vi "Connection State Callback.vi"(7 "Owner":refnum<class>, 8 "error in (no error)":errorcluster, 10 "Connection State":T1, 11 "Connection":refnum<class "Connection.lvclass">) -> (0 "error out":errorcluster)   [LabVIEW 2012, in "Chat Server.lvclass"]
uses:
  Chat Server.lvclass
  lv-stream/stream/Connection/Connection.lvclass
  lv-stream/stream/Connection State.ctl
  lv-stream/stream/Stream.lvlib
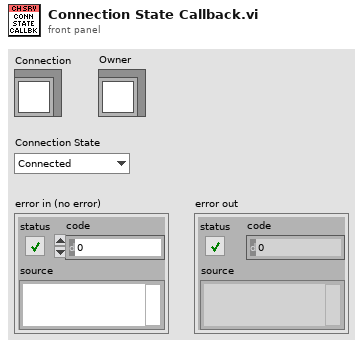
[diagram p1: front panel]
types:
  T1 = typedef "Stream.lvlib/Connection State.ctl" = enum16{"Connected", "Disconnected"}
  T2 = typedef "Chat Server.lvclass/Red Data.ctl" = cluster{"Connections":refnum<class "Connection.lvclass">[]}
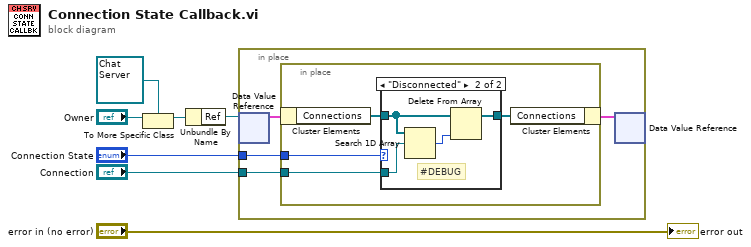
[diagram p0: block diagram]
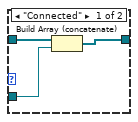
[diagram p2: hidden frame]
diagram:
  n1 = To More Specific Class(target class=refnum<class "Chat Server.lvclass"> refnum ("Chat Server.lvclass"), reference="Owner") -> (specific class reference=w4:refnum<class "Chat Server.lvclass">)  [unwired: 1 in, 1 out]
  n2 = Unbundle By Name(w4) -> ("Ref"=w5:refnum<data-value>)
  n3 = in-place {
    in-place-border: "Connection" -> [w9]
    in-place-border: "Connection State" -> [w8]
    n4 = in-place-dvr #1(w5) -> (w11:T2)  [unwired: 1 out]
    n5 = in-place {
      in-place-border: w9 -> [w13]
      in-place-border: w8 -> [w15]
      n6 = in-place-cluster #2(w11) -> ("Connections"=w14:refnum<class "Connection.lvclass">[])
      n7 = case shown="\"Disconnected\"" w15 {
        tunnel: w14 -> [w18 w21]
        tunnel: w13 -> [w17 w22]
        tunnel: [w16 w19] -> w12
        frame "Connected" {
          n8 = Build Array (concatenate)(w18, w17) -> (w16:refnum<class "Connection.lvclass">[])
        }
        frame "Disconnected" {
          # "#DEBUG"
          n9 = Search 1D Array(1D array=w21, element=w22) -> (index of element=w20:i32)  [unwired: 1 in]
          n10 = Delete From Array(array=w21, index=w20) -> (array with subset deleted=w19:refnum<class "Connection.lvclass">[])  [unwired: 1 in, 1 out]
        }
      }
      n11 = in-place-cluster #2("Connections"=w12) -> (w10:T2)
    }
    n12 = in-place-dvr #1(w10) -> ()  [unwired: 2 out]
  }
  "error out" <- "error in (no error)"
